vi "Hardware-DIB.vi"(8 "error in (no error)":errorcluster, 11 "DCM-DSI in":refnum<class "DCM-DSI.lvclass">) -> (0 "error out":errorcluster, 3 "DCM-DSI out":refnum<class "DCM-DSI.lvclass">)   [LabVIEW 2016, in "DSI-RT.lvlib"]
uses:
  DSI-RT.lvlib
  Classes/DCM-DSI/DCM-DSI.lvclass
  Classes/DCM-DSI/Read DCM Ref.vi
  Classes/DCM-DSI/Read DI-B Command.vi
  Classes/DCM-DSI/Read Pump-B Command.vi
  Classes/DCM-DSI/Write DI-B Command.vi
  Classes/DCM-DSI/Write Pump-B Command.vi
  <vilib>/Powertrain Controls/Device Drivers/DCM/Rev0/RT/DCM - RT.lvclass
  <vilib>/Powertrain Controls/Device Drivers/DCM/DI/RT/DCM - RT - DI.lvlib
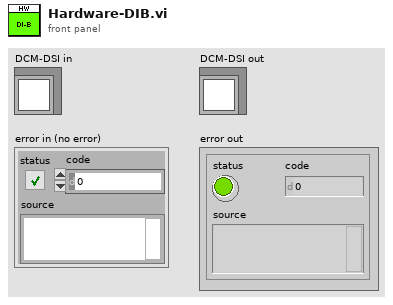
[diagram p1: front panel]
types:
  T1 = typedef "DCM - RT - DI.lvlib/Command.ctl" = cluster{"Mode":T2, "Digital Input":T3, "Default Profile Index":u8, "Cal Freq [Hz]":sgl, "Cal Duration [s]":sgl, "Cal Increment [s]":sgl, "Cal Pulses":u16, "TMP Command Sequence":T4[], "EPT TDC Offset [CAD]":sgl, "EPT Window Start [DBTDC]":sgl, "EPT Window End [DBTDC]":sgl, "EPT Angles":T5[], "EPT Skip Fire":bool, "EPT Skip Index":u8, "EPT Precharge Duration [s]":sgl, "EPT Precharge Profile Index":u8}
  T2 = typedef "DCM - FPGA - DI.lvlib/Mode.ctl" = enum8{"Off", "Direct", "Calibration", "Triggered Multi-Pulse", "Engine Position Tracking"}
  T3 = typedef "DCM - FPGA.lvlib/Digital Channel.ctl" = enum8{"Unused", "User OS", "Diff IO 1", "Diff IO 2", "Diff IO 3", "Diff IO 4", "Diff IO 5", "Diff IO 6", "Diff IO 7", "Diff IO 8", "Aux 1", "Aux 2", "Aux 3", "Aux 4", "Aux 5", "Aux 6", "Aux 7", "Aux 8", "Aux 9", "Aux 10", "Aux 11", "Aux 12", "Aux 13", "Aux 14", "Aux 15", "Aux 16"}
  T4 = typedef "DCM - RT - DI.lvlib/Command Sequence.ctl" = cluster{"Duration [s]":sgl, "Level":bool, "Run/Stop":bool, "Profile Index":u8}
  T5 = typedef "DCM - RT - DI.lvlib/Angle Control.ctl" = cluster{"Enable":bool, "Timing [DBTDC]":sgl, "Duration [s]":sgl, "Profile Index":u8}
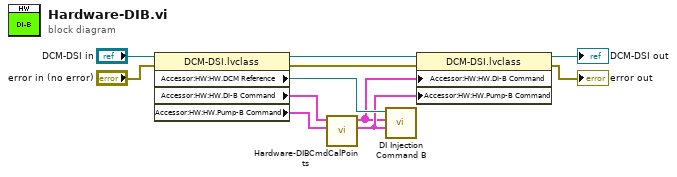
[diagram p0: block diagram]
diagram:
  n1 = property class="DCM-DSI.lvclass"(reference="DCM-DSI in", error in="error in (no error)") -> (reference out=w2:refnum<class "DCM-DSI.lvclass">, error out=w3:errorcluster, "Accessor:HW:HW.DCM Reference"=w11:refnum<class "DCM - RT.lvclass">, "Accessor:HW:HW.DI-B Command"=w7:T1[], "Accessor:HW:HW.Pump-B Command"=w6:T1)
  n2 = call "Hardware-DIBCmdCalPoints.vi"("Pump-B Command"=w6, "DI-B Command"=w7) -> ("Pump-B Command"=w10:T1, "DI-B Command"=w9:T1[])  [unwired: 6 in]
  n3 = call <vilib>:"DI Injection Command B.vi"("B Pump Command"=w10, "B DI Command"=w9, "DCM Reference"=w11) -> ()  [unwired: 9 in]
  n4 = property class="DCM-DSI.lvclass"(reference=w2, error in=w3, "Accessor:HW:HW.DI-B Command"=w9, "Accessor:HW:HW.Pump-B Command"=w10) -> (reference out=→"DCM-DSI out":refnum<class "DCM-DSI.lvclass">, error out=→"error out":errorcluster)
